vi "Traverse-Settings.vi"() -> ()   [LabVIEW 2016]
uses:
  TypeDefs/Trav-Settings-TD.ctl
  TypeDefs/Trav-Motion-TD.ctl
panel:
  in  "Settings":T1 {"Motion Type" items=["Linear", "Rotary"]}
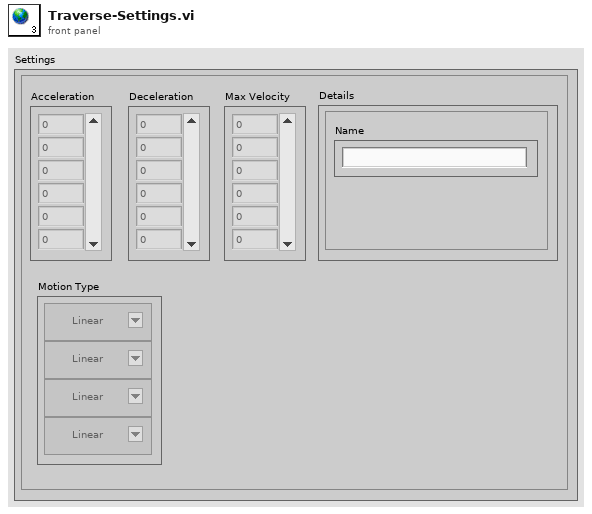
[diagram p1: front panel]
types:
  T1 = typedef "Trav-Settings-TD.ctl" = cluster{"Acceleration":dbl[], "Deceleration":dbl[], "Max Velocity":dbl[], "Details":cluster{"Name":string}, "Motion Type":T2[]}
  T2 = typedef "Trav-Motion-TD.ctl" = u16
diagram:
